vi "StartSequenceAcquisition.vi"(0 "Microscope in":refnum<class "Microscope.lvclass">, 5 "Exposure":i32=100, 7 "Frames":i32=100 caption="BufferSize", 9 "Interval":i32=100 caption="BufferSize", 11 "error in (no error)":errorcluster) -> (4 "Microscope out":refnum<class "Microscope.lvclass">, 15 "error out":errorcluster)   [LabVIEW 2020, in "Microscope.lvlib" / "Microscope.lvclass"]
uses:
  Microscope.lvclass
  Microscope.lvclass/Microscope.ctl
  Component/Camera/Camera Messages/StartSequenceAcqusition Msg/StartSequenceAcqusition Msg.lvclass/StartSequenceAcqusition Msg.ctl
  <vilib>/ActorFramework/Message Enqueuer/Message Enqueuer.lvclass/Message Enqueuer.ctl
  <vilib>/ActorFramework/Message Enqueuer/Enqueue.vi
  Component/Camera/Camera Messages/StartSequenceAcqusition Msg/StartSequenceAcqusition Msg.lvclass
  C:/Program Files/National Instruments/LabVIEW 2020/vi.lib/ActorFramework/Message/Message.lvclass
  <vilib>/ActorFramework/Message Priority Queue/Priority Enqueue.vi
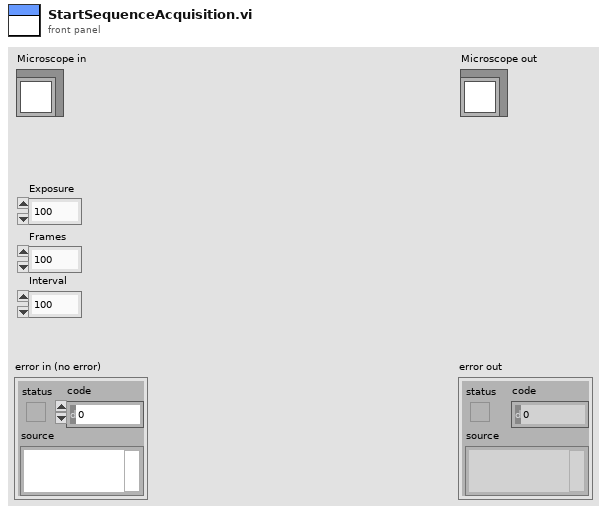
[diagram p1: front panel]
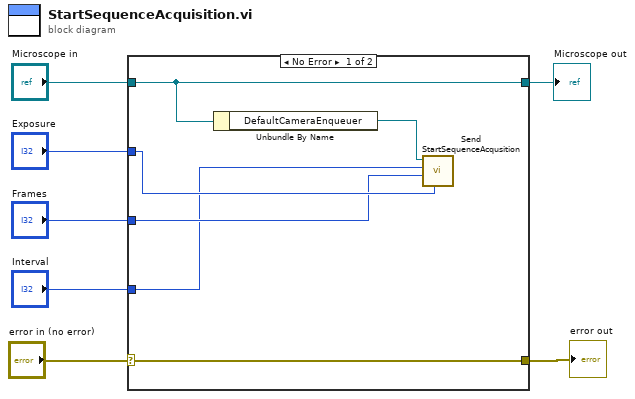
[diagram p0: block diagram]
diagram:
  n1 = case shown="No Error" "error in (no error)" {
    selector: "error in (no error)" -> [w8 w15]
    tunnel: [w8 w15] -> w6
    tunnel: "Microscope in" -> [w13 w14]
    tunnel: [w13 w14] -> w4
    tunnel: "Exposure" -> [w11 _]
    tunnel: "Frames" -> [w10 _]
    tunnel: "Interval" -> [w9 _]
    frame No Error {
      n2 = Unbundle By Name(w13) -> ("DefaultCameraEnqueuer"=w12:refnum<class "Message Enqueuer.lvclass">)
      n3 = call "Send StartSequenceAcqusition.vi"("Exposure"=w11, "Frames"=w10, "Interval"=w9, "Message Enqueuer"=w12) -> ()  [unwired: 6 in, 2 out]
    }
    frame Error {
    }
  }
  "error out" <- w6
  "Microscope out" <- w4
